vi "gxml_BldClusterAttr.vi"(3 "Num of Elements":i32) -> (1 "ClusterAttrString":string)   [LabVIEW 2011, in "Third Party VIs.lvlib" / "GXML.lvlib"]
uses:
  GXML.lvlib
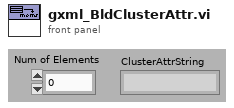
[diagram p1: front panel]
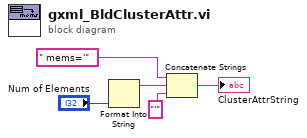
[diagram p0: block diagram]
diagram:
  n1 = Format Into String("Num of Elements") -> (resulting string=w4:string)  [unwired: 3 in, 1 out]
  n2 = Concatenate Strings(" mems='", w4, "'") -> (→"ClusterAttrString":string)
